vi "1D Fourier Series Experiment.vi"() -> ()   [LabVIEW 2020]
uses:
  <vilib>/Analysis/NI_AALBase.lvlib
panel:
  in  "Wave Table":dbl[](array[numeric])
  in  "Period":i32=1
  in  "Signal Type":enum16{"Sine Wave", "Square Wave", "Arbitrary"}(ring)
  out "Coefficients":cluster{"A0":dbl, "Am":dbl[], "Bm":dbl[]}
  in  "N":i32
  out "Signal":cluster{dbl, dbl, dbl[][]}(graph)
  in  "Signal Generation":T1={"samples"=128, "amplitude"=1.0, "phase(degrees)"=0.0, "cycles"=1.0} {"amplitude" format="%0.2f"; "cycles" format="%0.2f"; "phase(degrees)" format="%0.2f"}
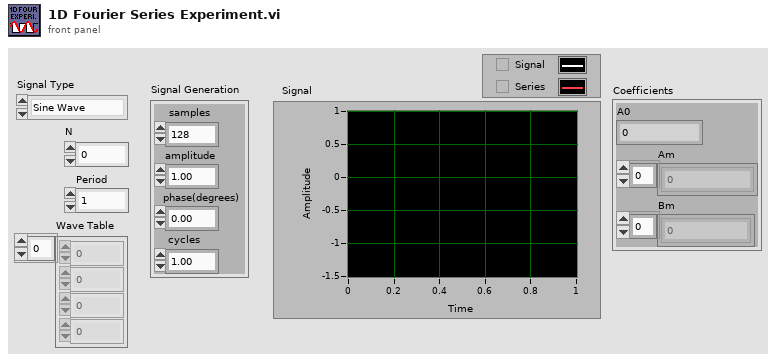
[diagram p1: front panel]
types:
  T1 = cluster{"samples":i32, "amplitude":dbl, "phase(degrees)":dbl, "cycles":dbl}
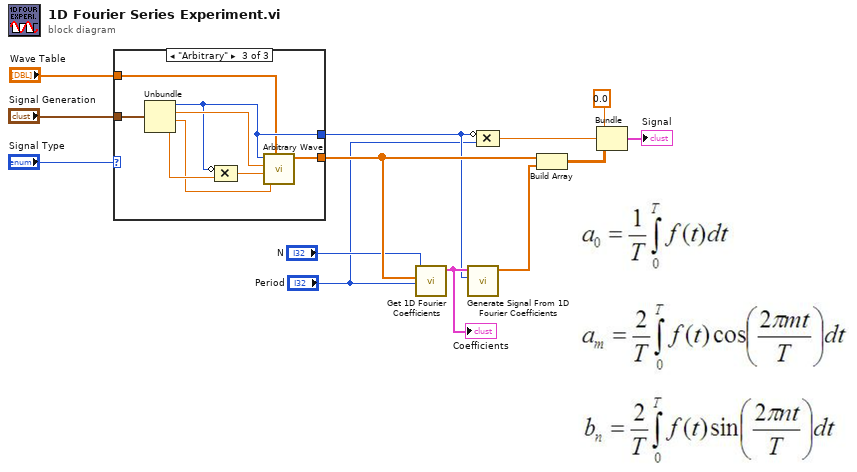
[diagram p0: block diagram]
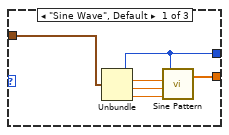
[diagram p2: hidden frame]
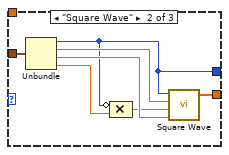
[diagram p3: hidden frame]
diagram:
  n1 = case shown="\"Arbitrary\"" "Signal Type" {
    tunnel: [w16 w26 w29] -> w9
    tunnel: [w15 w20 w28] -> w5
    tunnel: "Signal Generation" -> [w14 w25 w34]
    tunnel: "Wave Table" -> [_ _ w27]
    frame "Sine Wave", Default {
      n2 = Unbundle(w14) -> ("samples"=w15:i32, "amplitude"=w19:dbl, "phase(degrees)"=w18:dbl, "cycles"=w17:dbl)
      n3 = call <vilib>:"Sine Pattern.vi"("cycles"=w17, "phase(degrees)"=w18, "amplitude"=w19, "samples"=w15) -> ("Sinusoidal Pattern"=w16:dbl[])  [unwired: 1 out]
    }
    frame "Square Wave" {
      n4 = Unbundle(w25) -> ("samples"=w20:i32, "amplitude"=w24:dbl, "phase(degrees)"=w23:dbl, "cycles"=w22:dbl)
      n5 = Compound Arithmetic op=MULTIPLY(invert w20, w22) -> (w21:dbl)
      n6 = call <vilib>:"Square Wave.vi"("samples"=w20, "amplitude"=w24, "frequency"=w21, "phase in"=w23) -> ("square wave"=w26:dbl[])  [unwired: 2 in, 2 out]
    }
    frame "Arbitrary" {
      n7 = Unbundle(w34) -> ("samples"=w28:i32, "amplitude"=w31:dbl, "phase(degrees)"=w30:dbl, "cycles"=w32:dbl)
      n8 = Compound Arithmetic op=MULTIPLY(invert w28, w32) -> (w33:dbl)
      n9 = call <vilib>:"Arbitrary Wave.vi"("Wave Table"=w27, "phase in"=w30, "frequency"=w33, "amplitude"=w31, "samples"=w28) -> ("arbitrary wave"=w29:dbl[])  [unwired: 2 in, 2 out]
    }
  }
  n10 = call "Get 1D Fourier Coefficients.vi"("Period"="Period", "Signal"=w9, "#Coefficients"="N") -> ("Coefficients"=w6:cluster{"A0":dbl, "Am":dbl[], "Bm":dbl[]})  [unwired: 8 in]
  "Coefficients" <- w6
  n11 = call "Generate Signal From 1D Fourier Coefficients.vi"("Samples"=w5, "Coefficients in"=w6) -> ("Signal"=w7:dbl[])  [unwired: 9 in]
  n12 = Compound Arithmetic op=MULTIPLY(invert w5, "Period") -> (w11:dbl)
  n13 = Build Array(w9, w7) -> (w10:dbl[][])
  n14 = Bundle(0.0, w11, w10) -> (→"Signal":cluster{dbl, dbl, dbl[][]})  [unwired: 1 in]
